vi "test2-StateChange_Queue.vi"(8 "error in (no error)":errorcluster, 11 "TestCase in":refnum<class "testcase-CSMGlobalLog.lvclass">) -> (0 "error out":errorcluster, 3 "TestCase out":refnum<class "testcase-CSMGlobalLog.lvclass">)   [LabVIEW 2017, in "testcase-CSMGlobalLog.lvclass"]
uses:
  testcase-CSMGlobalLog.lvclass
  testcase-CSMGlobalLog.lvclass/testcase-CSMGlobalLog.ctl
  650155f4-1af1-443b-a877-8bdf29044e93.vi
  <vilib>/addons/_JKI Toolkits/VI Tester/TestCase.llb/TestCase.lvclass
  src/user.lib/_NEVSTOP/Communicable State Machine(CSM)/Utility/Periodic String Filter Setting.ctl
  src/user.lib/_NEVSTOP/Communicable State Machine(CSM)/Communicable State Machine.lvlib
  C:/Program Files (x86)/National Instruments/LabVIEW 2017/vi.lib/addons/_JKI Toolkits/VI Tester/TestCase.llb/TestCase.lvclass
panel:
  out "String cache total":string
  out "LoopCount":i32
  out "String Cache Each Loop":string
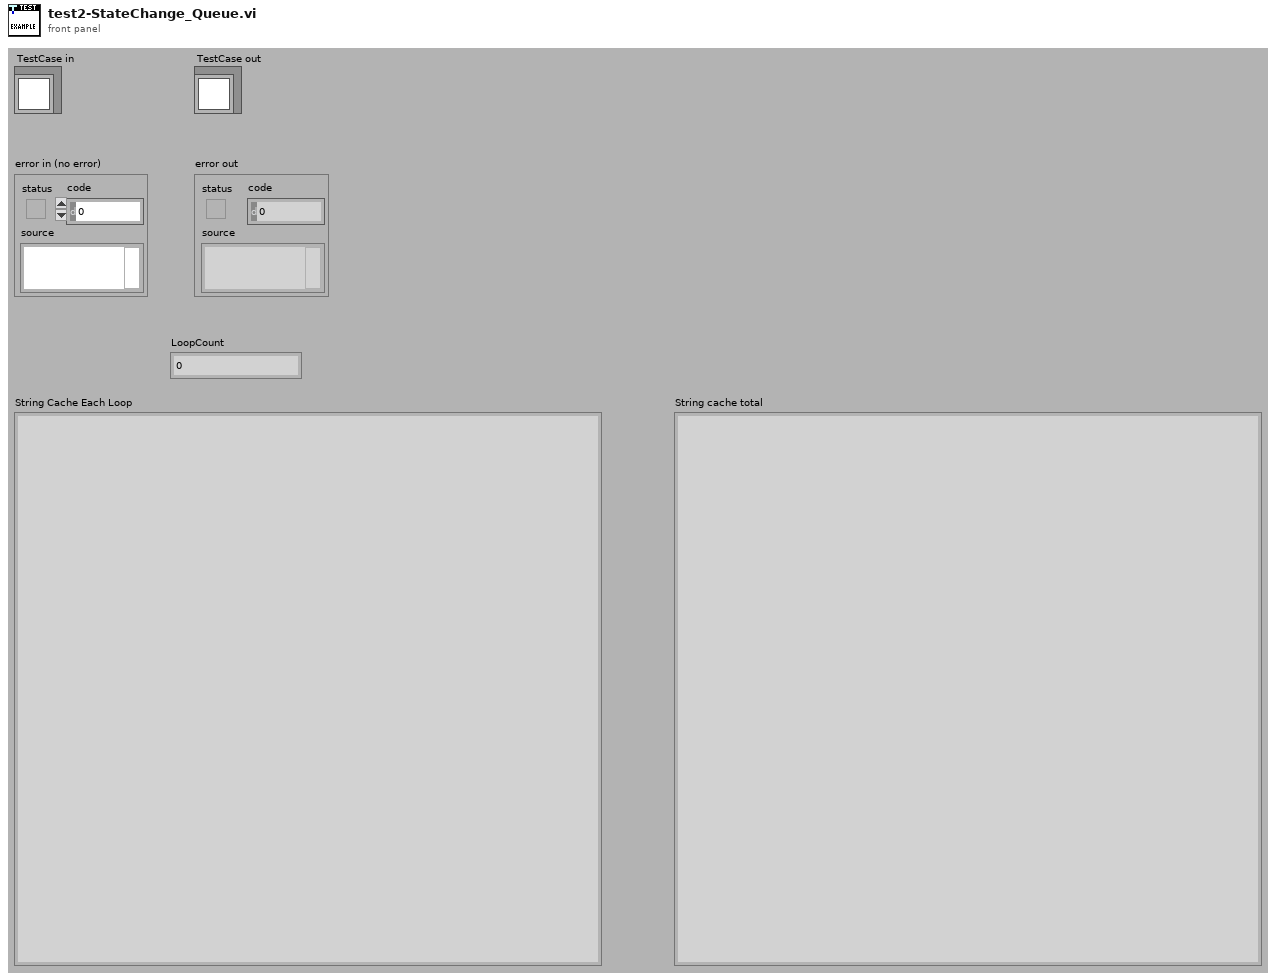
[diagram p1: front panel]
types:
  T1 = typedef "Communicable State Machine.lvlib/Periodic String Filter Setting.ctl" = cluster{"threashold(#/s)":dbl, "Check Peroid(s)":dbl}
  T2 = typedef "Communicable State Machine.lvlib/_CSM_GlobalLog_MSG.ctl" = cluster{"Name (\"\" to Use UUID)":string, "Current State":string, "Arguments":string, "Source Message":T3, "Source Module":string, "Complete(T)/Start(F)":bool, "LogType":T4, "Time Stamp":timestamp}
  T3 = typedef "Communicable State Machine.lvlib/_CSM_Response Source Message.ctl" = cluster{"‘State":string, "’Arguments":string, "’Error":errorcluster}
  T4 = typedef "Communicable State Machine.lvlib/_CSM_GlobalLog_MSG_TYPE.ctl" = enum16{"User Log", "State Change", "Status", "Interrupt", "Register", "Unregister", "Error Log", "Module Created", "Module Destroyed", "Async Message", "No-Rep Async Message", "Sync Message"}
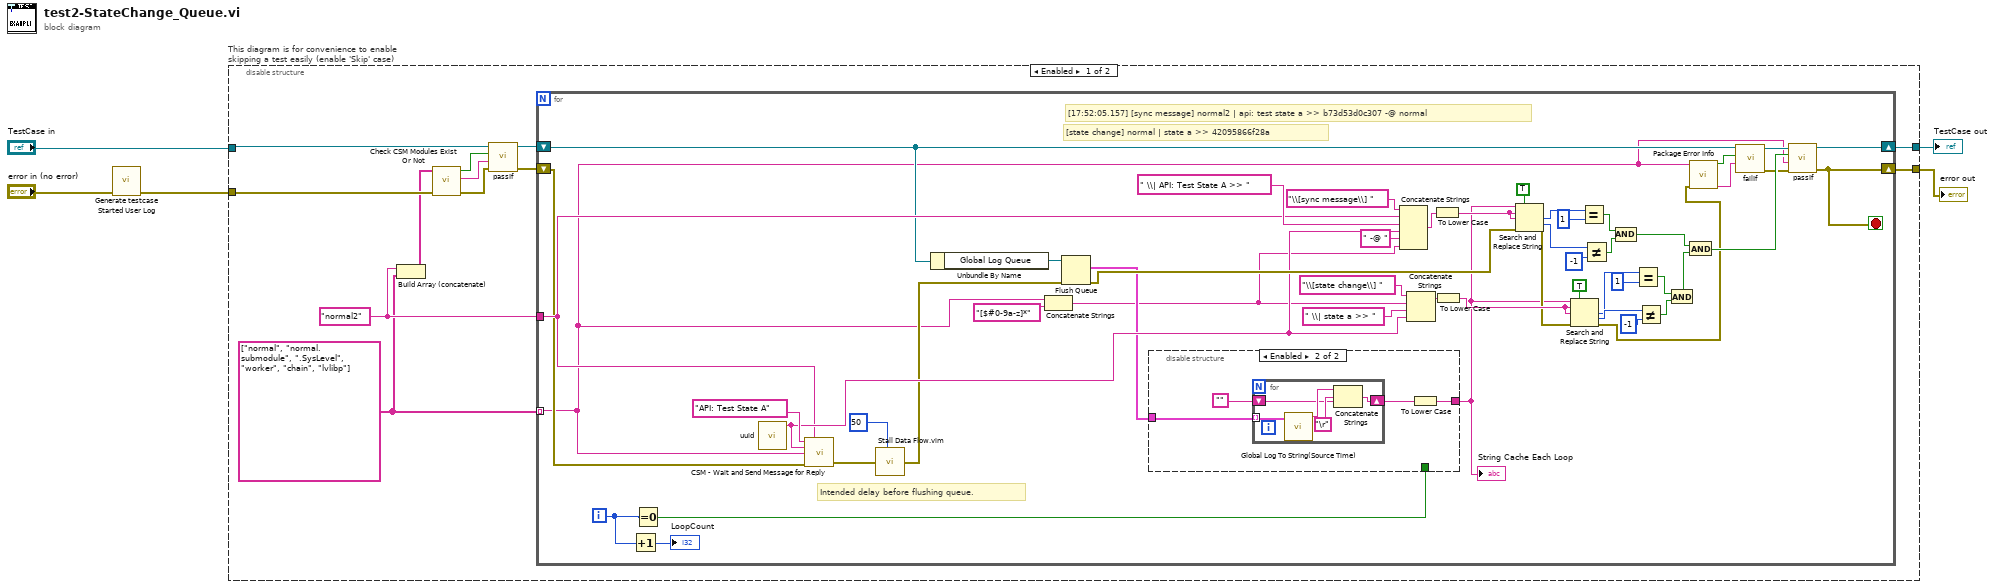
[diagram p0: block diagram]
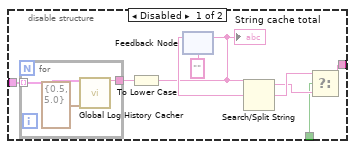
[diagram p2: hidden frame]
diagram:
  n1 = call "Generate testcase Started User Log.vi"("Error In"="error in (no error)") -> ("error out"=w1:errorcluster)  [unwired: 10 in]
  n2 = disable-structure "This diagram is for convenience to enable skipping a test easily (enable 'Skip' case)" shown="Enabled" {
    disable-tunnel: "TestCase in" -> [w12 w94]
    disable-tunnel: [w16 w92] -> w2
    disable-tunnel: [w17 w93] -> w4
    disable-tunnel: w1 -> [w9 w91]
    frame Enabled {
      w8 = "normal2" ("CSM")
      w7 = string[] ["normal", "normal.submodule", ".SysLevel", "worker", "chain", "lvlibp"]
      n3 = Build Array (concatenate)(w8, w7) -> (w6:string[])
      n4 = call "Check CSM Modules Exist Or Not.vi"("error in"=w9, "CSM names in"=w6) -> ("error out"=w13:errorcluster, "Debug string"=w14:string, "All Modules Exist?"=w15:bool)  [unwired: 7 in]
      n5 = call-dynamic "passIf.vi"("error in (no error)"=w13, "message (\"\")"=w14, "pass"=w15, "TestCase in"=w12) -> ("error out"=w10:errorcluster, "TestCase out"=w11:refnum<class "testcase-CSMGlobalLog.lvclass">)  [unwired: 6 in]
      n6 = for {
        tunnel: w7 -> [w18] mode=indexing
        shift-right: [w37] -> w17
        shift-left: w10 -> [w25]
        shift-right: [w69] -> w16
        shift-left: w11 -> [w20]
        tunnel: w8 -> [w27]
        i -> [w29]
        stop <- w37 stop-if-true
        # "[17:52:05.157] [sync message] normal2 | api: test state a >> b73d53d0c307 -@ normal"
        # "Intended delay before flushing queue."
        # "[state change] normal | state a >> 42095866f28a"
        n7 = Increment(x=w29) -> (x+1=→"LoopCount":i32)
        n8 = Equal To 0?(x=w29) -> (x = 0?=w28:bool)
        n9 = call "uuid.vi"() -> ("UUID"=w40:string)  [unwired: 11 in]
        n10 = call "CSM - Wait and Send Message for Reply.vi"("State"="API: Test State A", "Current Module (\"\" to Generate an ID)"=w27, "Arguments (\"\")"=w40, "Target Module"=w18, "Error In (No Error)"=w25) -> ("error out"=w34:errorcluster)  [unwired: 7 in, 3 out]
        n11 = call "Stall Data Flow.vim"("value in"=w34, "milliseconds to wait"=u32 50) -> ("value out"=w33:errorcluster)  [unwired: 1 out]
        n12 = Unbundle By Name(w20) -> ("Global Log Queue"=w68:refnum<queue>)
        n13 = Concatenate Strings(w18, "[$#0-9a-z]*" ("string")) -> (w26:string)
        n14 = Flush Queue(queue=w68, error in (no error)=w33) -> (remaining elements=w31:T2[], error out=w46:errorcluster)  [unwired: 1 out]
        n15 = disable-structure shown="Enabled" {
          disable-tunnel: [w72 w82] -> w30
          disable-tunnel: w28 -> [w71 _]
          disable-tunnel: w31 -> [w70 w84]
          frame Disabled {
            n16 = for {
              tunnel: w70 -> [w81] mode=indexing
              tunnel: [w80] -> w78
              n17 = call "Global Log History Cacher.vi"("Global Log Data"=w81, "Settings"=T1 {"threashold(#/s)"=0.5, "Check Peroid(s)"=5.0}) -> ("String Cache"=w80:string)  [unwired: 13 in]
            }
            n18 = To Lower Case(string=w78) -> (all lower case string=w73:string)
            "String cache total" <- w73
            n19 = feedback #1("") -> (w77:string)
            n20 = feedback-in #1(w73) -> ()
            n21 = Search/Split String(string=w73, search string/char (-)=w77) -> (substring before match=w74:string, match + rest of string=w75:string)  [unwired: 1 in, 1 out]
            n22 = Select(t=w75, s=w71, f=w74) -> (s? t:f=w72:string)
          }
          frame Enabled {
            n23 = for {
              tunnel: w84 -> [w90] mode=indexing
              shift-right: [w86] -> w83
              shift-left: "" -> [w87]
              n24 = call "Global Log To String(Source Time).vi"("Log"=w90) -> ("Log String"=w89:string)  [unwired: 9 in]
              n25 = Concatenate Strings(w89, "\r", w87) -> (w86:string)
            }
            n26 = To Lower Case(string=w83) -> (all lower case string=w82:string)
          }
        }
        "String Cache Each Loop" <- w30
        n27 = Concatenate Strings("\\[sync message\\] " ("regular expression"), w27, " \\| API: Test State A >> " ("string"), w40, " -@ " ("string"), w26) -> (w63:string)
        n28 = Concatenate Strings("\\[state change\\] " ("regular expression"), w26, " \\| state a >> " ("string"), w40) -> (w65:string)
        n29 = To Lower Case(string=w63) -> (all lower case string=w61:string)
        n30 = To Lower Case(string=w65) -> (all lower case string=w49:string)
        n31 = Search and Replace String(replace all?=TRUE ("replace all? (F)"), input string=w30, search string=w61, replace string=w61, error in=w46) -> (number of replacements=w60:i32, offset past replacement=w59:i32, error out=w48:errorcluster)  [unwired: 3 in, 1 out]
        n32 = Search and Replace String(replace all?=TRUE ("replace all? (F)"), input string=w30, search string=w49, replace string=w49, error in=w48) -> (number of replacements=w51:i32, offset past replacement=w52:i32, error out=w19:errorcluster)  [unwired: 3 in, 1 out]
        n33 = Equal?(x=w60, y=1) -> (x = y?=w57:bool)
        n34 = Not Equal?(x=w59, y=-1) -> (x != y?=w56:bool)
        n35 = And(x=w57, y=w56) -> (x .and. y?=w38:bool)
        n36 = Equal?(x=w51, y=1) -> (x = y?=w54:bool)
        n37 = Not Equal?(x=w52, y=-1) -> (x != y?=w55:bool)
        n38 = And(x=w54, y=w55) -> (x .and. y?=w47:bool)
        n39 = And(x=w38, y=w47) -> (x .and. y?=w35:bool)
        n40 = call "Package Error Info.vi"("error in"=w19, "String in"=w18) -> ("packed error info out"=w23:string, "error status"=w24:bool)  [unwired: 8 in]
        n41 = call-dynamic "failIf.vi"("message (\"\")"=w23, "fail"=w24, "TestCase in"=w20) -> ("error out"=w21:errorcluster, "TestCase out"=w22:refnum<class "testcase-CSMGlobalLog.lvclass">)  [unwired: 7 in]
        n42 = call-dynamic "passIf.vi"("error in (no error)"=w21, "message (\"\")"=w18, "pass"=w35, "TestCase in"=w22) -> ("error out"=w37:errorcluster, "TestCase out"=w69:refnum<class "testcase-CSMGlobalLog.lvclass">)  [unwired: 6 in]
      }
    }
    frame Disabled {
      # "skip test result while test is under development"
      n43 = call <vilib>:"skip.vi"("error in (no error)"=w91, "TestCase in"=w94) -> ("error out"=w93:errorcluster, "TestCase out"=w92:refnum<class "testcase-CSMGlobalLog.lvclass">)  [unwired: 8 in]
    }
  }
  "error out" <- w4
  "TestCase out" <- w2
